vi "MB Ethernet Slave Ingen control de variables.vi"() -> ()   [LabVIEW 2017, in "Lib_Esclavo_Ingen.lvlib"]
uses:
  Lib_Esclavo_Ingen.lvlib
panel:
  out "000001":bool
  out "400001":u16
  out "Input Registers":u16[](array[numeric])
  out "Consumo eléctrico Isla Numblar":u16[](array[numeric])
  in  "Stop":bool
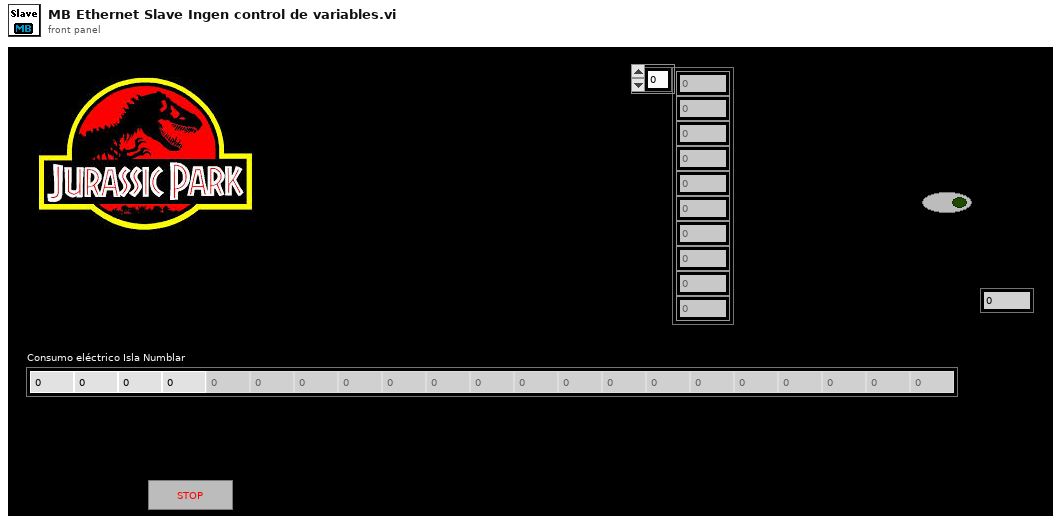
[diagram p1: front panel]
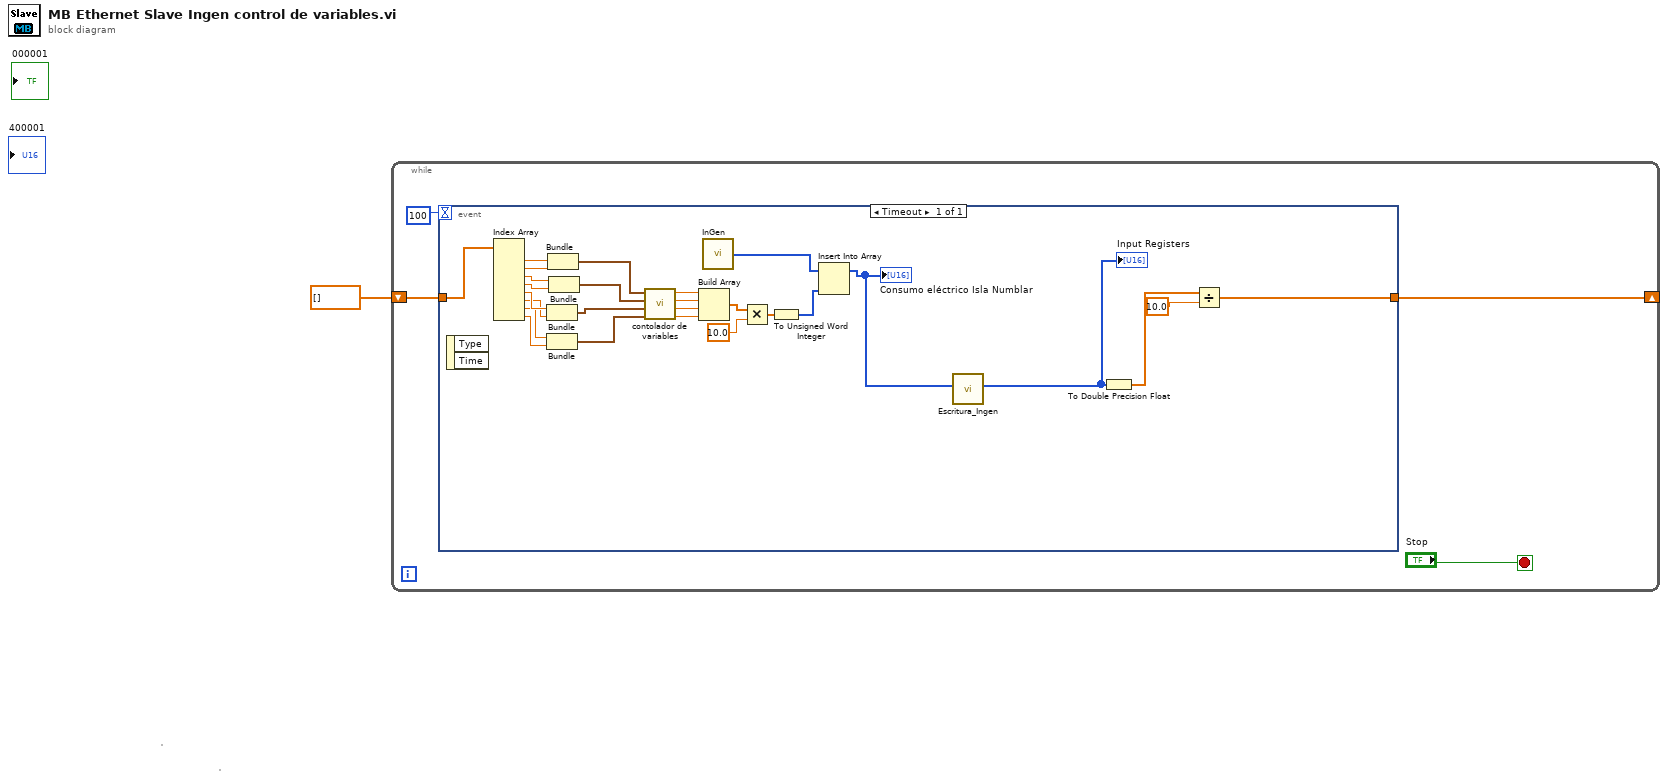
[diagram p0: block diagram]
diagram:
  n1 = while {
    shift-right: [w4] -> _
    shift-left: dbl[] [] -> [w3]
    stop <- "Stop" stop-if-true
    n2 = event shown="[0] Timeout" {
      selector: _ -> [_]
      dyn-events: _ -> [_]
      timeout: 100 -> [_]
      tunnel: [w21] -> w4
      tunnel: w3 -> [w20]
      event Timeout {
        n3 = event-data() -> ()  [unwired: 3 out]
        n4 = Index Array(array=w20) -> (element #1=w19:dbl, element #2=w18:dbl, element #3=w17:dbl, element #4=w16:dbl, element #5=w15:dbl, element #6=w14:dbl, element #7=w13:dbl, element #8=w12:dbl)  [unwired: 8 in]
        n5 = Bundle(w15, w14) -> (w9:cluster{dbl, dbl})  [unwired: 1 in]
        n6 = Bundle(w13, w12) -> (w8:cluster{dbl, dbl})  [unwired: 1 in]
        n7 = Bundle(w19, w18) -> (w11:cluster{dbl, dbl})  [unwired: 1 in]
        n8 = Bundle(w17, w16) -> (w10:cluster{dbl, dbl})  [unwired: 1 in]
        n9 = call "contolador de variables.vi"("CONTROL DE LLENADO"=w8, "CONTROL DE HUMEDAD"=w9, "CONTROL DE PRESIÓN"=w10, "CONTROL TEMPERATURA"=w11) -> ("VOLUMEN ACTUAL"=w29:dbl, "HUMEDAD ACTUAL"=w30:dbl, "PRESIÓN ACTUAL"=w31:dbl, "TEMPERATURA ACTUAL"=w32:dbl)  [unwired: 4 in]
        n10 = Build Array(w32, w31, w30, w29) -> (w28:dbl[])
        n11 = call "InGen.vi"() -> ("Variables de planta"=w25:u16[])
        n12 = Multiply(x=w28, y=10.0 ("VOLUMEN ACTUAL")) -> (x*y=w26:dbl[])
        n13 = To Unsigned Word Integer(number=w26) -> (unsigned 16bit integer=w24:u16[])
        n14 = Insert Into Array(array=w25, new element=w24) -> (w7:u16[])  [unwired: 1 in]
        "Consumo eléctrico Isla Numblar" <- w7
        n15 = call "Escritura_Ingen.vi"("Entrada_Variables"=w7) -> ("Escritura_Variabes"=w6:u16[])  [unwired: 10 in]
        "Input Registers" <- w6
        n16 = To Double Precision Float(number=w6) -> (double precision float=w23:dbl[])
        n17 = Divide(x=w23, y=10.0) -> (x/y=w21:dbl[])
      }
    }
  }
